vi "JSONRPC-Info.vi"(8 "error in (no error)":errorcluster, 11 "info":string) -> (0 "error out":errorcluster, 3 "result":string)   [LabVIEW 2014]
doc: "Invokes the actual implementation of a RIP <b>method</b>."
uses:
  Configuration/Global_Configurations.vi
panel:
  # "Info"
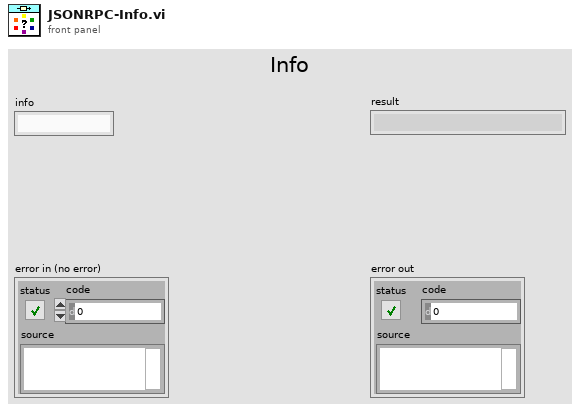
[diagram p1: front panel]
types:
  T1 = enum16{"POST_SET", "POST_GET", "SSE_GET", "GET_INFO"}
  T2 = cluster{"Path":path, "Name":string, "Authors":string, "Keywords":string, "Description":string, "Cameras":cluster{"Base URL":string, "Path":string, "Name":string}[]}[]
  T3 = cluster{"Name":string, "Type":string, "Min":string, "Max":string, "Precision":string, "Description":string}[]
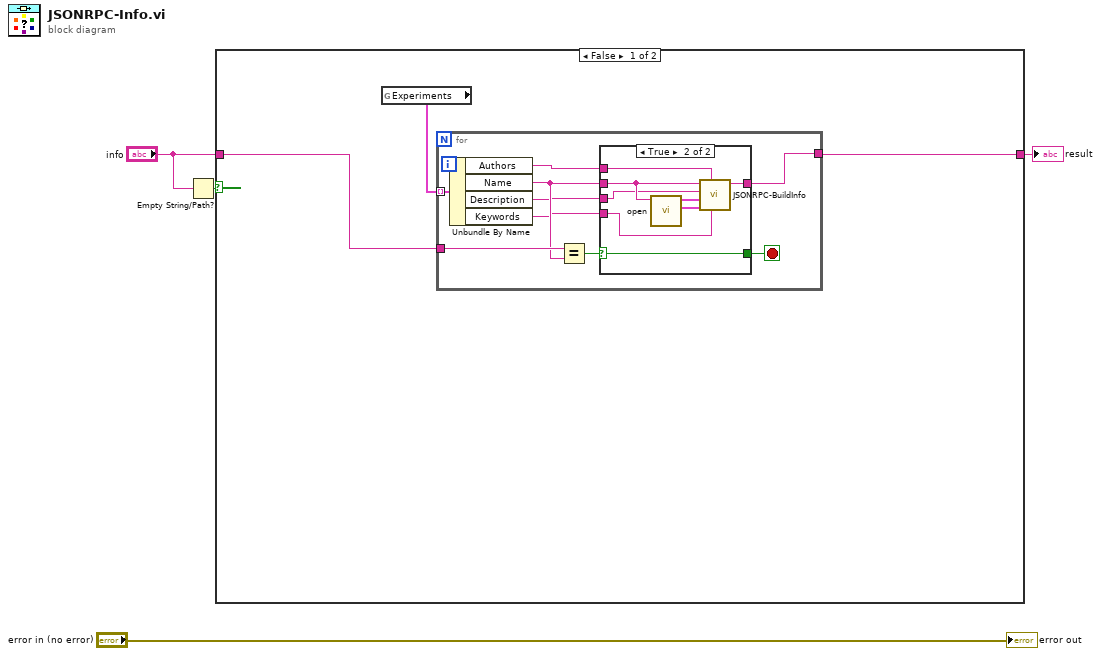
[diagram p0: block diagram]
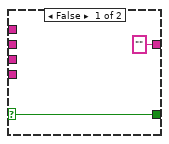
[diagram p2: hidden frame]
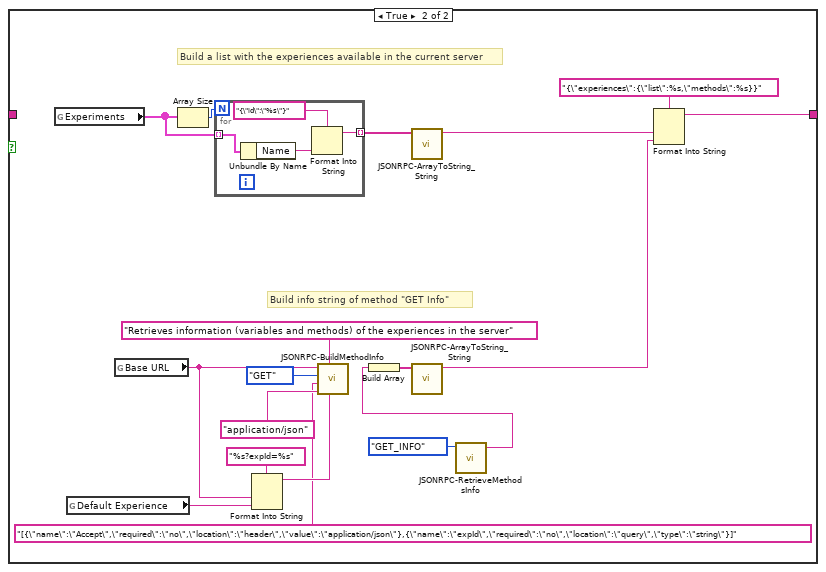
[diagram p3: hidden frame]
diagram:
  n1 = Empty String/Path?(string/path="info") -> (empty?=w3:bool)
  n2 = case shown="False" w3 {
    tunnel: "info" -> [w6 _]
    tunnel: [w5 w27] -> w1
    frame False {
      n3 = global read "Global_Configurations.vi" "Experiments"() -> (w7:T2)
      n4 = for {
        tunnel: w7 -> [w16] mode=indexing
        tunnel: w6 -> [w15]
        tunnel: [w8] -> w5
        stop <- w12 stop-if-true
        n5 = Unbundle By Name(w16) -> ("Authors"=w11:string, "Name"=w14:string, "Description"=w10:string, "Keywords"=w9:string)
        n6 = Equal?(x=w15, y=w14) -> (x = y?=w13:bool)
        n7 = case shown="True" w13 {
          selector: w13 -> [w17 w22]
          tunnel: w14 -> [_ w24]
          tunnel: w10 -> [_ w21]
          tunnel: w9 -> [_ w19]
          tunnel: w11 -> [_ w20]
          tunnel: ["" ("info") w23] -> w8
          tunnel: [w17 w22] -> w12
          frame False {
          }
          frame True {
            n8 = call "open.vi"("Experience ID"=w24) -> ("Indicators_list"=w26:T3, "Controls_list"=w25:T3)  [unwired: 8 in, 1 out]
            n9 = call "JSONRPC-BuildInfo.vi"("keywords"=w19, "authors"=w20, "readables"=w26, "writables"=w25, "description"=w21, "expId"=w24) -> ("info"=w23:string)  [unwired: 5 in]
          }
        }
      }
    }
    frame True {
      # "Build a list with the experiences available in the current server"
      # "Build info string of method \"GET Info\""
      n10 = global read "Global_Configurations.vi" "Experiments"() -> (w43:T2)
      n11 = global read "Global_Configurations.vi" "Default Experience"() -> (w41:string)
      n12 = global read "Global_Configurations.vi" "Base URL"() -> (w40:string)
      n13 = Array Size(array=w43) -> (size(s)=w44:i32)
      n14 = for {
        N: w44 -> [_]
        tunnel: w43 -> [w48] mode=indexing
        tunnel: [w45] -> w33 mode=indexing
        n15 = Unbundle By Name(w48) -> ("Name"=w47:string)
        n16 = Format Into String(format string="{\"id\":\"%s\"}", w47) -> (resulting string=w45:string)  [unwired: 2 in, 1 out]
      }
      n17 = Format Into String(format string="%s?expId=%s", w40, w41) -> (resulting string=w39:string)  [unwired: 2 in, 1 out]
      n18 = call "JSONRPC-BuildMethodInfo.vi"("Example"=w39, "Description"="Retrieves information (variables and methods) of the experiences in the server", "Returns"="application/json", "Params"="[{\"name\":\"Accept\",\"required\":\"no\",\"location\":\"header\",\"value\":\"application/json\"},{\"name\":\"expId\",\"required\":\"no\",\"location\":\"query\",\"type\":\"string\"}]", "Method"=enum16{"SSE", "GET", "POST"}."GET", "url"=w40) -> ()  [unwired: 5 in, 1 out]
      n19 = call "JSONRPC-ArrayToString_String.vi"("Array"=w33) -> ("Output"=w32:string)  [unwired: 10 in]
      n20 = call "JSONRPC-RetrieveMethodsInfo.vi"("Method"=T1."GET_INFO") -> ("Output"=w28:string)  [unwired: 10 in]
      n21 = Build Array(w28) -> (w42:string[])
      n22 = call "JSONRPC-ArrayToString_String.vi"("Array"=w42) -> ("Output"=w34:string)  [unwired: 10 in]
      n23 = Format Into String(format string="{\"experiences\":{\"list\":%s,\"methods\":%s}}" ("Description"), w32, w34) -> (resulting string=w27:string)  [unwired: 2 in, 1 out]
    }
  }
  "result" <- w1
  "error out" <- "error in (no error)"
